vi "Find Element.vi"(0 "Variant (Cluster) in":variant, 7 "Name":string, 11 "error in (no error)":errorcluster) -> (4 "Variant (Cluster) out":variant, 6 "element":variant, 8 "found?":bool, 10 "index of element":i32, 15 "error out":errorcluster)   [LabVIEW 2017, in "Advanced Variant Tools.lvlib"]
uses:
  Advanced Variant Tools.lvlib
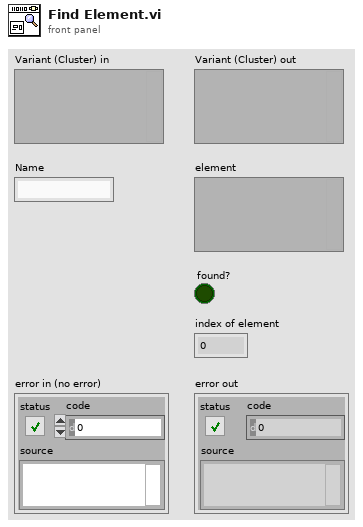
[diagram p1: front panel]
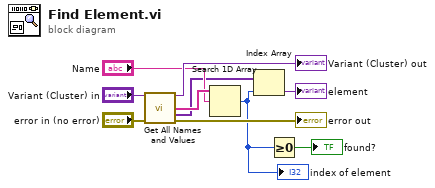
[diagram p0: block diagram]
diagram:
  n1 = call "Get All Names and Values.vi"("Variant (Cluster) In"="Variant (Cluster) in", "error in"="error in (no error)") -> ("Variant (Cluster) Out"=→"Variant (Cluster) out":variant, "Element Names"=w8:string[], "Values"=w5:variant[], "error out"=→"error out":errorcluster)  [unwired: 9 in, 1 out]
  n2 = Search 1D Array(1D array=w8, element="Name") -> (index of element=w2:i32)  [unwired: 1 in]
  "index of element" <- w2
  n3 = Index Array(array=w5, index=w2) -> (element=→"element":variant)
  n4 = Greater Or Equal To 0?(x=w2) -> (x >= 0?=→"found?":bool)
